vi "Convert Type Code.vi"(1 "pvxs type code":u8) -> (0 "type code":T1)   [LabVIEW 2020, in "PV Access.lvlib" / "PV Data.lvlib" / "PV Data.lvclass"]
uses:
  PV Data.lvclass
  Type Code.ctl
  PV Data.lvlib
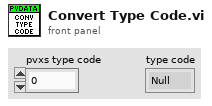
[diagram p1: front panel]
types:
  T1 = typedef "PV Access.lvlib/PV Data.lvlib/Type Code.ctl" = enum8{"Null", "Bool", "BoolA", "Int8", "Int8A", "Int16", "Int16A", "Int32", "Int32A", "Int64", "Int64A", "UInt8", "UInt8A", "UInt16", "UInt16A", "UInt32", "UInt32A", "UInt64", "UInt64A", "Float32", "Float32A", "Float64", "Float64A", "String", "StringA", "Struct", "StructA", "Union", "UnionA", "Any", "AnyA"}
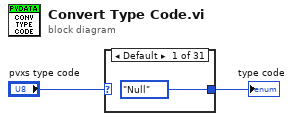
[diagram p0: block diagram]
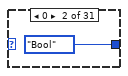
[diagram p2: hidden frame]
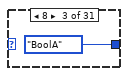
[diagram p3: hidden frame]
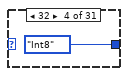
[diagram p4: hidden frame]
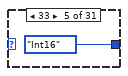
[diagram p5: hidden frame]
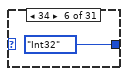
[diagram p6: hidden frame]
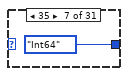
[diagram p7: hidden frame]
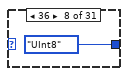
[diagram p8: hidden frame]
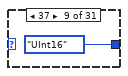
[diagram p9: hidden frame]
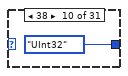
[diagram p10: hidden frame]
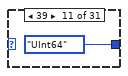
[diagram p11: hidden frame]
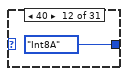
[diagram p12: hidden frame]
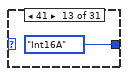
[diagram p13: hidden frame]
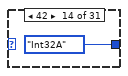
[diagram p14: hidden frame]
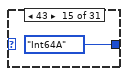
[diagram p15: hidden frame]
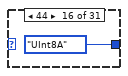
[diagram p16: hidden frame]
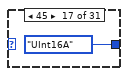
[diagram p17: hidden frame]
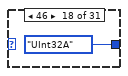
[diagram p18: hidden frame]
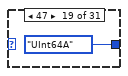
[diagram p19: hidden frame]
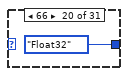
[diagram p20: hidden frame]
diagram:
  n1 = case shown="Default" "pvxs type code" {
    tunnel: [Type_Code."Null" ("type code") Type_Code."Bool" ("type code") Type_Code."BoolA" ("type code") Type_Code."Int8" ("type code") Type_Code."Int16" ("type code") Type_Code."Int32" ("type code") Type_Code."Int64" ("type code") Type_Code."UInt8" ("type code") Type_Code."UInt16" ("type code") Type_Code."UInt32" ("type code") Type_Code."UInt64" ("type code") Type_Code."Int8A" ("type code") Type_Code."Int16A" ("type code") Type_Code."Int32A" ("type code") Type_Code."Int64A" ("type code") Type_Code."UInt8A" ("type code") Type_Code."UInt16A" ("type code") Type_Code."UInt32A" ("type code") Type_Code."UInt64A" ("type code") Type_Code."Float32" ("type code") Type_Code."Float64" ("type code") Type_Code."Float32A" ("type code") Type_Code."Float64A" ("type code") Type_Code."String" ("type code") Type_Code."StringA" ("type code") Type_Code."Struct" ("type code") Type_Code."Union" ("type code") Type_Code."Any" ("type code") Type_Code."StructA" ("type code") Type_Code."UnionA" ("type code") Type_Code."AnyA" ("type code")] -> w1
    frame Default {
    }
    frame 0 {
    }
    frame 8 {
    }
    frame 32 {
    }
    frame 33 {
    }
    frame 34 {
    }
    frame 35 {
    }
    frame 36 {
    }
    frame 37 {
    }
    frame 38 {
    }
    frame 39 {
    }
    frame 40 {
    }
    frame 41 {
    }
    frame 42 {
    }
    frame 43 {
    }
    frame 44 {
    }
    frame 45 {
    }
    frame 46 {
    }
    frame 47 {
    }
    frame 66 {
    }
    frame 67 {
    }
    frame 74 {
    }
    frame 75 {
    }
    frame 96 {
    }
    frame 104 {
    }
    frame 128 {
    }
    frame 129 {
    }
    frame 130 {
    }
    frame 136 {
    }
    frame 137 {
    }
    frame 138 {
    }
  }
  "type code" <- w1
